vi "Grouped_Proj _newa_steploop_FINAL_tabs.vi"() -> ()   [LabVIEW 2017]
uses:
  <instrlib>/Lake Shore 336/Public/Data/Sensor Data (Single Reading).vi
  <vilib>/Utility/file.llb/Read Delimited Spreadsheet (DBL).vi
  <vilib>/Utility/file.llb/Write Delimited Spreadsheet (DBL).vi
  <instrlib>/Lake Shore 336/Lake Shore 336.lvlib
panel:
  in  "Tab Control":enum32{"Controlls", "Graphs"}(tab)
  in  "Source Meter address":refnum<visa-resource-name>="GPIB1::29::INSTR"
  out "Measured Resistance (Ohms)":dbl format="%#_6p"
  in  "Resistance Range Lower Limit (2 Ohm)":dbl=2.0 format="%#_6p"
  in  "Resistance Range Upper Limit (2E+8 Ohm)":dbl=200000000.0 format="%#_6p"
  in  "Resistance NPLC (0.1)":dbl=0.1
  in  "Resistance Range (2 Ohm)":dbl=2.0
  in  "Resistance Auto Range (T: Enable)":bool=TRUE
  in  "file to save data (dialog if empty)":path
  in  "Temperature controller address":refnum<visa-resource-name>
  out "Measured Temperature":dbl format="%.6p"
  in  "Output's Control Loop (1:1)":u16(ring)=1 items=["1"=1, "2"=2]
  in  "Input (0:None)":u16(ring) items=["None", "A", "B", "C", "D"]
  in  "Mode (0:Off)":u16(ring) items=["Off", "Closed Loop PID", "Zone", "Open Loop"]
  in  "Max Current":u16(ring) items=["User Specified", "0.707 A", "1.0 A", "1.141 A", "2.0 A"]
  in  "Gain (P) (50.0)":dbl=50.0 format="%.1f"
  in  "Reset (I) (20.0)":dbl=20.0 format="%.1f"
  in  "Rate (D) (0.0 %)":dbl format="%.1f"
  in  "Manual Output (0.00 %)":dbl format="%.2f"
  in  "Range (0:Off)":u16(ring) items=["Off", "Low (On)", "Medium", "High"]
  in  "Temp start":dbl
  in  "step":dbl
  in  "Temp end":dbl
  in  "Temp tolerance":dbl
  out "R T Graph":cluster{"all rows":dbl[], "all rows":dbl[]}(graph)
  in  "stop":bool
  in  "Error In":errorcluster
  # "Resistance vs Temperature Measurement (Step mode)"
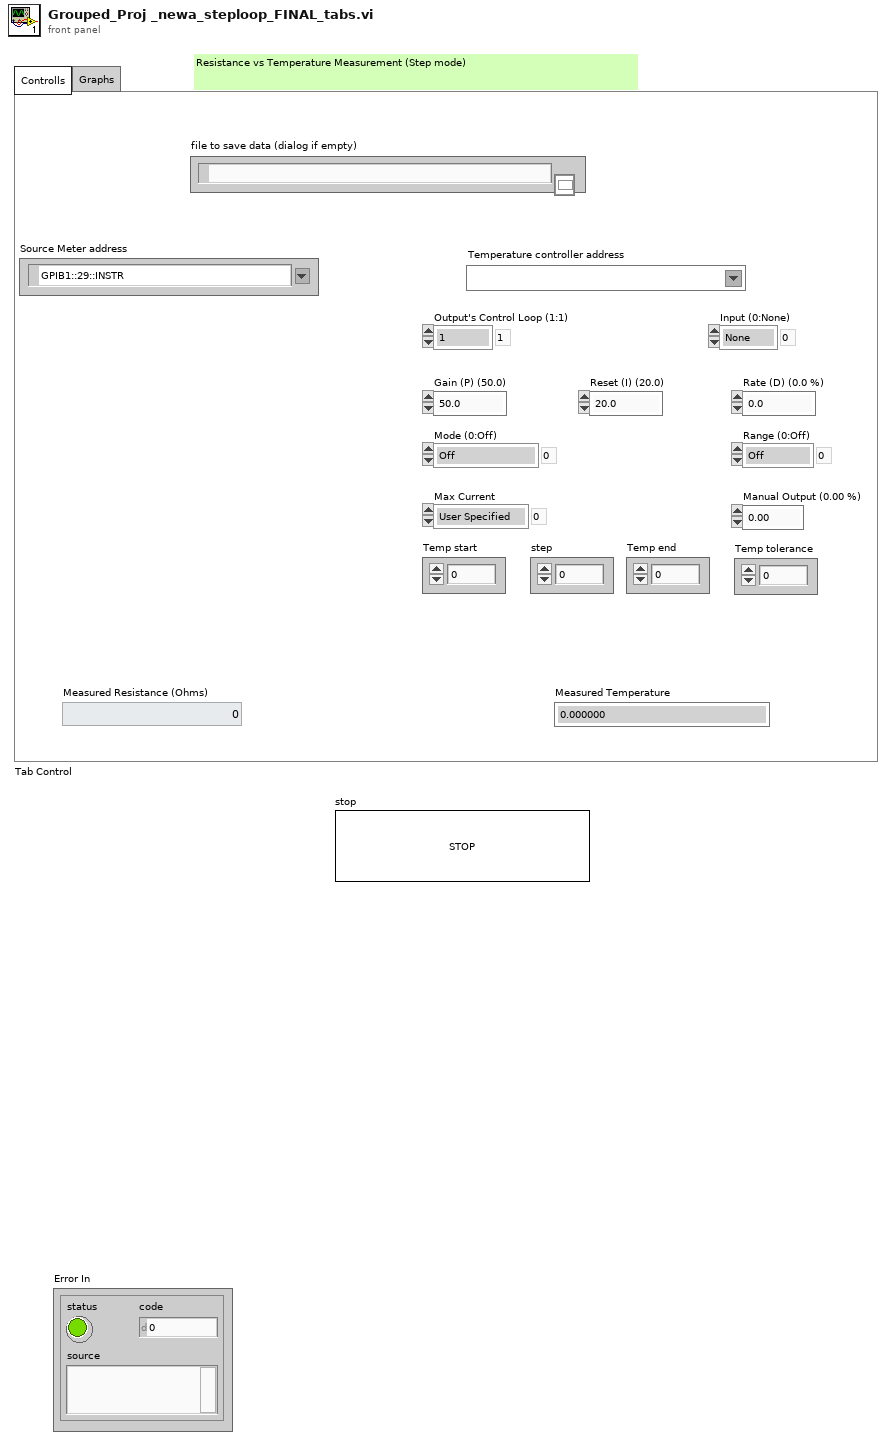
[diagram p1: front panel]
types:
  T1 = cluster{"Baud Rate":u32, "Parity":u16, "Data Bits":u16, "Stop Bits":u16, "Flow Control":u16}
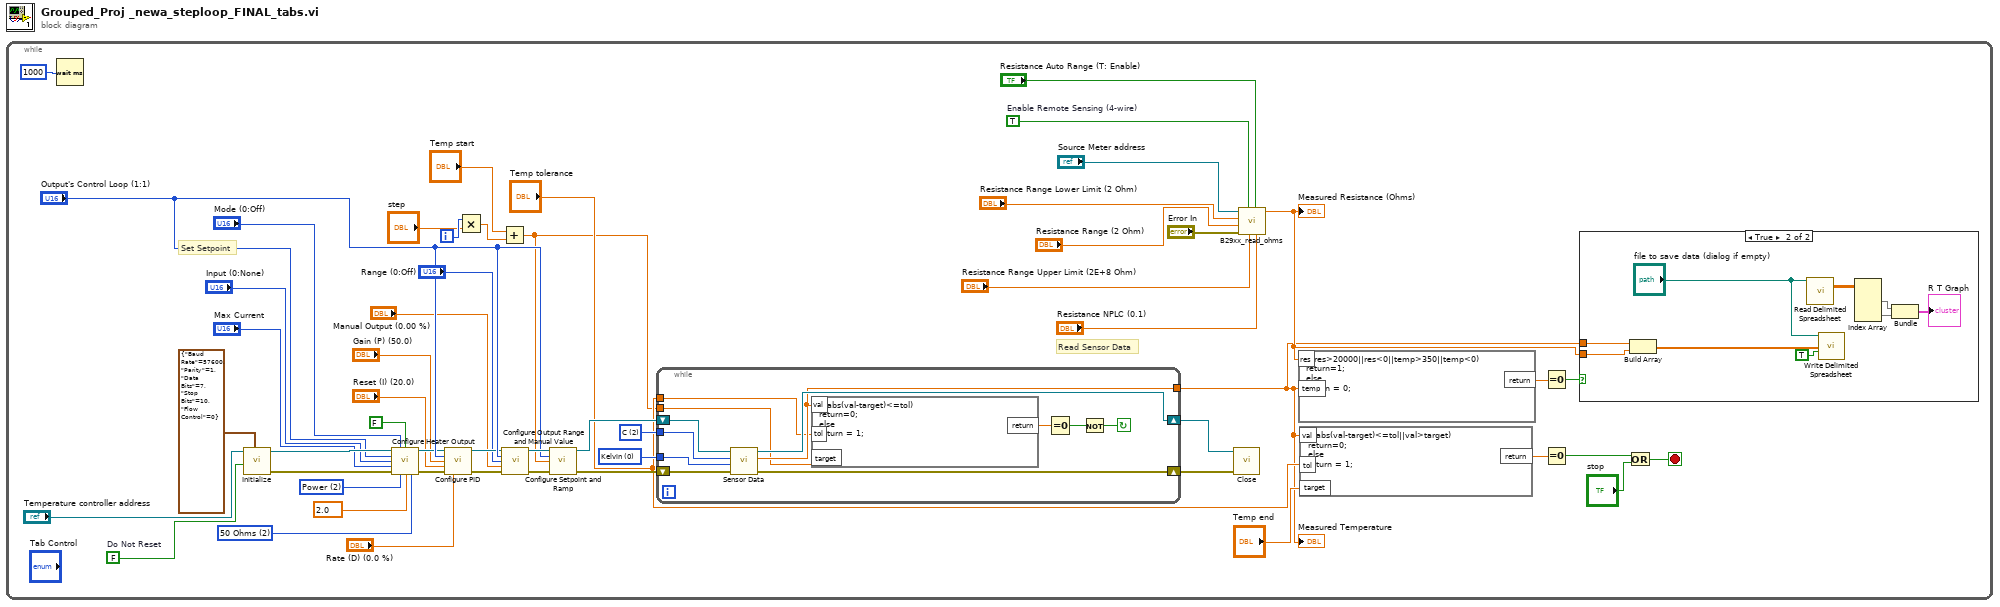
[diagram p0: block diagram]
diagram:
  n1 = while {
    i -> [w9]
    stop <- w14 stop-if-true
    w17 = u16 2 items=["A", "B", "C", "D"] ("Input (0:A)")
    w24 = u16 2 items=["50 Ohms"=2, "25 Ohms"=1] ("Heater Resistance (default to 50Ohms)")
    w37 = u16 0 items=["Kelvin", "Celsius", "Sensor Units"] ("Data Source (0:Kelvin)")
    w26 = u16 2 items=["Current"=1, "Power"=2] ("Heater Out Display (1:Current)")
    w41 = FALSE  # Do Not Reset
    w52 = TRUE  # Enable Remote Sensing (4-wire)
    # "Set Setpoint"
    # "Read Sensor Data"
    n2 = Wait (ms)(milliseconds to wait=u32 1000) -> ()  [unwired: 1 out]
    n3 = call <instrlib>:"Initialize.vi"("Serial Configuration"=T1 {"Baud Rate"=57600, "Parity"=1, "Data Bits"=7, "Stop Bits"=10, "Flow Control"=0}, "Reset (True)"=w41, "VISA resource name"="Temperature controller address") -> ("error out"=w45:errorcluster, "VISA resource name out"=w46:refnum<visa-resource-name>)  [unwired: 7 in]
    n4 = call <instrlib>:"Configure Heater Output.vi"("VISA resource name"=w46, "Mode (0:Off)"="Mode (0:Off)", "Power Up Enable (F: Off)"=FALSE, "Heater Output (1:1)"="Output's Control Loop (1:1)", "Input (0:None)"="Input (0:None)", "Max Current (0:User Specified)"="Max Current", "error in (no error)"=w45, "Heater Out Display (1:Current)"=w26, "Max User Current (2.000)"=2.0, "Heater Resistance (1:25 Ohms)"=w24) -> ("VISA resource name out"=w32:refnum<visa-resource-name>, "error out"=w33:errorcluster)  [unwired: 4 in]
    n5 = call <instrlib>:"Configure PID.vi"("VISA resource name"=w32, "Output's Control Loop (1:1)"="Output's Control Loop (1:1)", "Gain (P) (50.0)"="Gain (P) (50.0)", "Reset (I) (20.0)"="Reset (I) (20.0)", "error in (no error)"=w33, "Rate (D) (0.0 %)"="Rate (D) (0.0 %)") -> ("VISA resource name out"=w31:refnum<visa-resource-name>, "error out"=w30:errorcluster)  [unwired: 8 in]
    n6 = Multiply(x=w9, y="step") -> (x*y=w7:dbl)
    n7 = Add(x="Temp start", y=w7) -> (x+y=w5:dbl)
    n8 = call <instrlib>:"Configure Output Range and Manual Value.vi"("VISA resource name"=w31, "Output (1:1)"="Output's Control Loop (1:1)", "Range (0:Off)"="Range (0:Off)", "Manual Output (0.00 %)"="Manual Output (0.00 %)", "error in (no error)"=w30) -> ("VISA resource name out"=w43:refnum<visa-resource-name>, "error out"=w42:errorcluster)  [unwired: 9 in]
    n9 = call <instrlib>:"Configure Setpoint and Ramp.vi"("VISA resource name"=w43, "Output's Control Loop (1:1)"="Output's Control Loop (1:1)", "Setpoint (0.00000)"=w5, "error in (no error)"=w42) -> ("VISA resource name out"=w39:refnum<visa-resource-name>, "error out"=w38:errorcluster)  [unwired: 10 in]
    n10 = while {
      tunnel: w37 -> [w73]
      tunnel: w17 -> [w70]
      tunnel: [w68] -> w1
      shift-right: [w72] -> w36
      shift-left: w39 -> [w75]
      shift-right: [w71] -> w35
      shift-left: w38 -> [w74]
      tunnel: "Temp tolerance" -> [w67]
      tunnel: w5 -> [w66]
      stop <- w64 continue-if-true
      n11 = call-poly <instrlib>:"Sensor Data.vi"("error in (no error)"=w74, "Data Source (0:Kelvin)"=w73, "Input (0:A)"=w70, "VISA resource name"=w75) -> ("error out"=w71:errorcluster, "Sensor Data"=w68:dbl, "VISA resource name out"=w72:refnum<visa-resource-name>)  [unwired: 5 in]
      n12 = formula code="if(abs(val-target)<=tol)\nreturn=0;\nelse \nreturn = 1;"("val"=w68, "tol"=w67, "target"=w66) -> ("return"=w69:dbl)
      n13 = Equal To 0?(x=w69) -> (x = 0?=w65:bool)
      n14 = Not(x=w65) -> (.not. x?=w64:bool)
    }
    "Measured Temperature" <- w1
    n15 = call <instrlib>:"Close.vi"("error in (no error)"=w35, "VISA resource name"=w36) -> ()  [unwired: 9 in, 1 out]
    n16 = call "B29xx_read_ohms.vi"("Resistance NPLC (0.1)"="Resistance NPLC (0.1)", "Resistance Auto Range (T: Enable)"="Resistance Auto Range (T: Enable)", "Resistance Range Upper Limit (2E+8 Ohm)"="Resistance Range Upper Limit (2E+8 Ohm)", "Enable Remote Sensing (4-wire)"=w52, "error in (no error)"="Error In", "Resistance Range (2 Ohm)"="Resistance Range (2 Ohm)", "Resistance Range Lower Limit (2 Ohm)"="Resistance Range Lower Limit (2 Ohm)", "VISA Refnum in"="Source Meter address") -> ("Measurement Result"=w2:dbl)  [unwired: 2 in, 1 out]
    "Measured Resistance (Ohms)" <- w2
    n17 = formula code="if(res>20000||res<0||temp>350||temp<0)\nreturn=1;\nelse \nreturn = 0;"("res"=w2, "temp"=w1) -> ("return"=w4:dbl)
    n18 = formula code="if(abs(val-target)<=tol||val>target)\nreturn=0;\nelse \nreturn = 1;"("val"=w1, "tol"="Temp tolerance", "target"="Temp end") -> ("return"=w12:dbl)
    n19 = Equal To 0?(x=w4) -> (x = 0?=w3:bool)
    n20 = Equal To 0?(x=w12) -> (x = 0?=w13:bool)
    n21 = case shown="True" w3 {
      tunnel: w2 -> [_ w60]
      tunnel: w1 -> [_ w61]
      frame False {
      }
      frame True {
        n22 = Build Array(w61, w60) -> (w62:dbl[])
        n23 = call-poly <vilib>:"Read Delimited Spreadsheet.vi"("file path (dialog if empty)"="file to save data (dialog if empty)") -> ("all rows"=w56:dbl[][])  [unwired: 9 in, 5 out]
        n24 = call-poly <vilib>:"Write Delimited Spreadsheet.vi"("file path (dialog if empty)"="file to save data (dialog if empty)", "1D data"=w62, "append to file? (new file:F)"=TRUE) -> ()  [unwired: 11 in, 2 out]
        n25 = Index Array(array=w56) -> (element #1=w57:dbl[], element #2=w58:dbl[])  [unwired: 4 in]
        n26 = Bundle("all rows"=w57, "all rows"=w58) -> (→"R T Graph":cluster{"all rows":dbl[], "all rows":dbl[]})  [unwired: 1 in]
      }
    }
    n27 = Or(x=w13, y="stop") -> (x .or. y?=w14:bool)
  }
